vi "WSD Responce Bytes Count.vi"() -> (0 "Bytes Count":u32)   [LabVIEW 2016, in "Samwontech TEMP2xxx.lvlib"]
uses:
  <instrlib>/Samwontech TEMP2xxx/Samwontech TEMP2xxx.lvlib
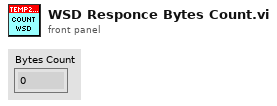
[diagram p1: front panel]
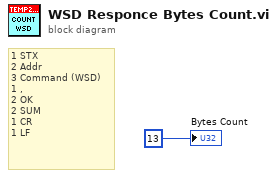
[diagram p0: block diagram]
diagram:
  # "1 STX\n2 Addr\n3 Command (WSD)\n1 ,\n2 OK\n2 SUM\n1 CR\n1 LF"
  "Bytes Count" <- u32 13
